vi "Operate-on-array.vi"(1 "Comparator value":dbl, 2 "Operateur":bool caption="greater then ? (flase if lower then)", 3 "Array-to-shrink":dbl[](array[numeric])) -> (0 "Shrinked-Array":dbl[](array[numeric]))   [LabVIEW 2011]
panel:
  out "index":dbl
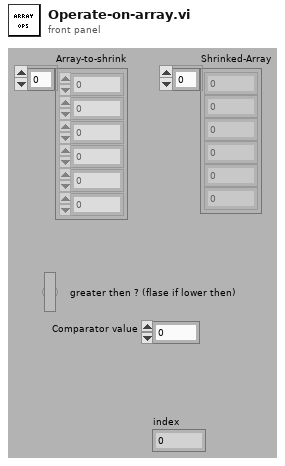
[diagram p1: front panel]
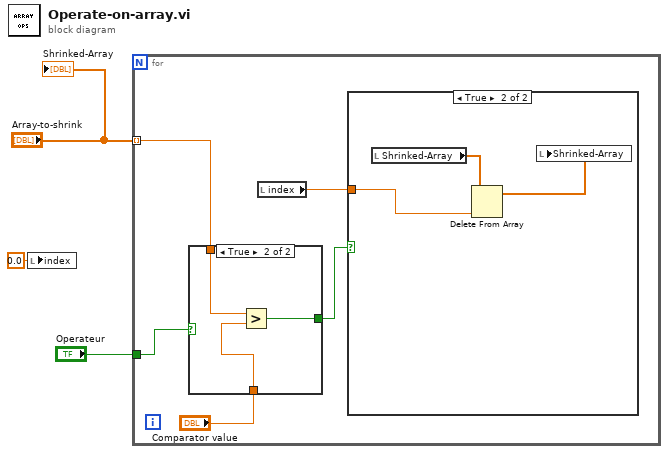
[diagram p0: block diagram]
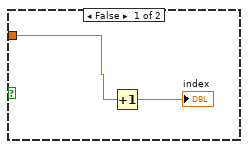
[diagram p2: hidden frame]
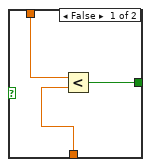
[diagram p3: hidden frame]
diagram:
  n1 = local write "index"(0.0 ("index")) -> ()
  n2 = for {
    tunnel: "Operateur" -> [w8]
    tunnel: "Array-to-shrink" -> [w6] mode=indexing
    n3 = case shown="True" w8 {
      tunnel: "Comparator value" -> [w16 w19]
      tunnel: w6 -> [w15 w18]
      tunnel: [w14 w17] -> w5
      frame False {
        n4 = Less?(x=w15, y=w16) -> (x < y?=w14:bool)
      }
      frame True {
        n5 = Greater?(x=w18, y=w19) -> (0:w17:bool)
      }
    }
    n6 = local read "index"() -> (w4:dbl)
    n7 = case shown="True" w5 {
      tunnel: w4 -> [w9 w11]
      frame False {
        n8 = Increment(x=w9) -> (x+1=→"index":dbl)
      }
      frame True {
        n9 = local read "Shrinked-Array"() -> (w13:dbl[])
        n10 = Delete From Array(array=w13, index=w11) -> (array with subset deleted=w12:dbl[])  [unwired: 1 in, 1 out]
        n11 = local write "Shrinked-Array"(w12) -> ()
      }
    }
  }
  "Shrinked-Array" <- "Array-to-shrink"
